vi "Auto_Routine_Deposit_Balance.vi"(8 "error in (no error)":errorcluster, 10 "Game Piece":T1, 11 "Position":T2=enum."Middle") -> (0 "error out":errorcluster)   [LabVIEW 2020]
uses:
  Arm/ArmPositionPreset.ctl
  Arm/ArmGamePiecePreset.ctl
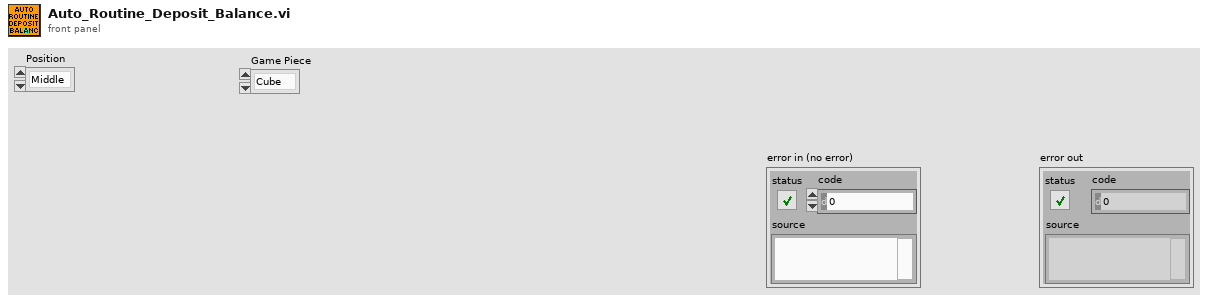
[diagram p1: front panel]
types:
  T1 = typedef "ArmGamePiecePreset.ctl" = enum16{"Cube", "Cone"}
  T2 = typedef "ArmPositionPreset.ctl" = enum16{"Upper", "Lower", "Middle", "Home", "Shelf", "Floor"}
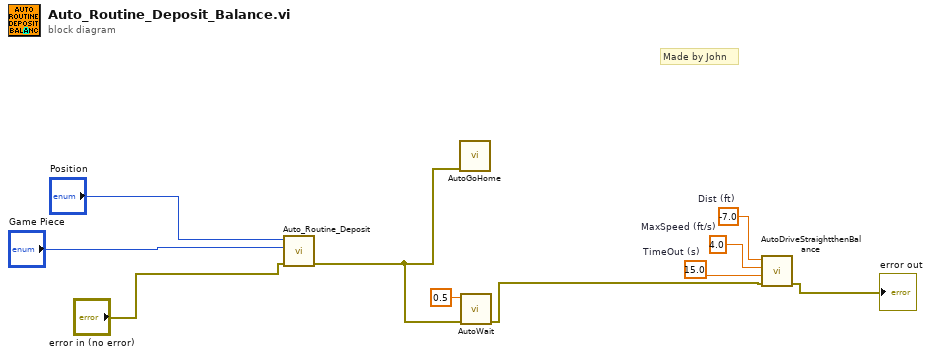
[diagram p0: block diagram]
diagram:
  w8 = 15.0  # TimeOut (s)
  w9 = 4.0  # MaxSpeed (ft/s)
  w10 = -7.0  # Dist (ft)
  # "Made by John"
  n1 = call "Auto_Routine_Deposit.vi"("error in (no error)"="error in (no error)", "Game Piece"="Game Piece", "Position"="Position") -> ("error out"=w2:errorcluster)  [unwired: 8 in]
  n2 = call "AutoGoHome.vi"("error in (no error)"=w2) -> ()  [unwired: 10 in, 1 out]
  n3 = call "AutoWait.vi"("error in (no error)"=w2, "TimeOut (s)"=0.5) -> ("error out"=w1:errorcluster)  [unwired: 9 in]
  n4 = call "AutoDriveStraightthenBalance.vi"("error in (no error)"=w1, "TimeOut (s)"=w8, "MaxSpeed (ft/s)"=w9, "Dist (ft)"=w10) -> ("error out"=→"error out":errorcluster)  [unwired: 7 in]
